vi "Set Delay.vi"(8 "error in (no error)":errorcluster, 9 "channel (1)":u8=1 min=1 max=4 step=1, 10 "delay (0 s)":dbl=0.5 min=0.0 max=32.767 format="%.3f", 11 "VISA resource name":refnum<visa-resource-name>) -> (0 "error out":errorcluster, 3 "VISA resource name out":refnum<visa-resource-name>)   [LabVIEW 2020, in "Agilent 6XXX Series.lvlib"]
doc: "This function sets the delay feature of the instrument."
uses:
  <instrlib>/Agilent 6XXX Series/Agilent 6XXX Series.lvlib
panel:
  # "*662xA only"
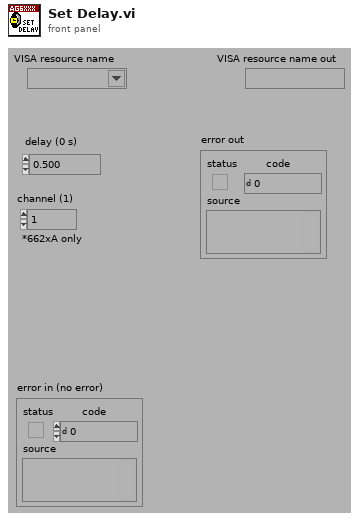
[diagram p1: front panel]
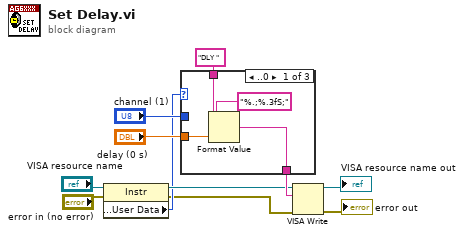
[diagram p0: block diagram]
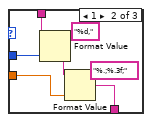
[diagram p2: hidden frame]
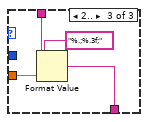
[diagram p3: hidden frame]
diagram:
  n1 = property class="Instr"(reference="VISA resource name", error in="error in (no error)") -> (reference out=w5:refnum<visa-resource-name>, error out=w1:errorcluster, "General Settings:User Data"=w2:u32)
  n2 = case shown="..0" w2 {
    tunnel: "DLY " -> [w14 w21 w25]
    tunnel: "delay (0 s)" -> [w13 w17 w24]
    tunnel: "channel (1)" -> [_ w22 _]
    tunnel: [w12 w16 w23] -> w6
    frame ..0 {
      n3 = Format Value(string ("")=w14, format string="%.;%.3fS;", value (0)=w13) -> (output string=w12:string)
    }
    frame 1 {
      n4 = Format Value(string ("")=w21, format string="%d,", value (0)=w22) -> (output string=w18:string)
      n5 = Format Value(string ("")=w18, format string="%.;%.3f;", value (0)=w17) -> (output string=w16:string)
    }
    frame 2.. {
      n6 = Format Value(string ("")=w25, format string="%.;%.3f;", value (0)=w24) -> (output string=w23:string)
    }
  }
  n7 = VISA Write(VISA resource name=w5, write buffer=w6, error in (no error)=w1) -> (VISA resource name out=→"VISA resource name out":refnum<visa-resource-name>, error out=→"error out":errorcluster)  [unwired: 1 out]
